vi "SUB-module-초를 문자열로 변환1.vi"(1 "입력-초단위":dbl) -> (0 "시:분:초":string)   [LabVIEW 2015]
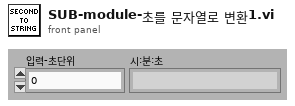
[diagram p1: front panel]
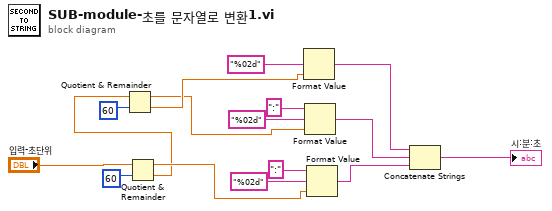
[diagram p0: block diagram]
diagram:
  n1 = Quotient & Remainder(x="입력-초단위", y=u16 60) -> (x-y*floor(x/y)=w11:dbl, floor(x/y)=w8:dbl)
  n2 = Quotient & Remainder(x=w8, y=u16 60) -> (x-y*floor(x/y)=w1:dbl, floor(x/y)=w4:dbl)
  n3 = Format Value(format string="%02d", value (0)=w4) -> (output string=w3:string)  [unwired: 1 in]
  n4 = Format Value(string ("")=":", format string="%02d", value (0)=w1) -> (output string=w2:string)
  n5 = Format Value(string ("")=":", format string="%02d", value (0)=w11) -> (output string=w10:string)
  n6 = Concatenate Strings(w3, w2, w10) -> (→"시:분:초":string)
